vi "Segment_b.vi"(11 "Input in Binary":bool[](array[boolean])) -> (3 "Segment b":bool)   [LabVIEW 2024]
panel:
  out "D":bool
  out "C":bool
  out "B":bool
  out "A":bool
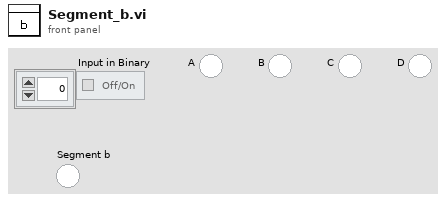
[diagram p1: front panel]
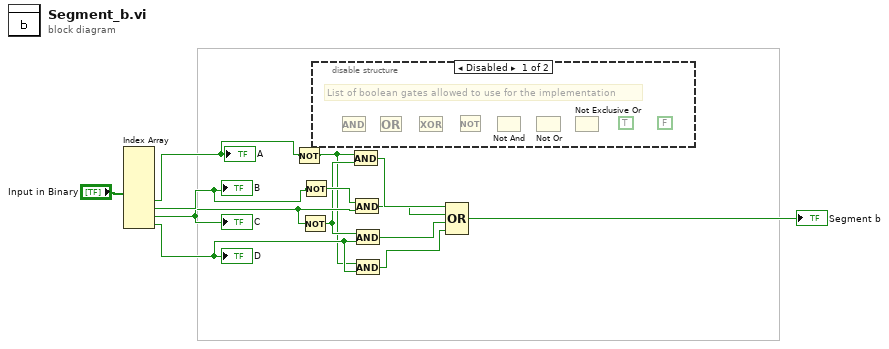
[diagram p0: block diagram]
diagram:
  n1 = Index Array(array="Input in Binary") -> (element #5=w9:bool, element #6=w12:bool, element #7=w10:bool, element #8=w7:bool)  [unwired: 8 in, 4 out]
  "A" <- w9
  "B" <- w12
  "C" <- w10
  "D" <- w7
  n2 = Not(x=w9) -> (.not. x?=w6:bool)
  n3 = Not(x=w10) -> (.not. x?=w8:bool)
  n4 = Not(x=w12) -> (.not. x?=w11:bool)
  n5 = disable-structure shown="Disabled" {
    frame Disabled {
      (unwired) FALSE
      (unwired) TRUE
      # "List of boolean gates allowed to use for the implementation"
      n6 = And() -> ()  [unwired: 2 in, 1 out]
      n7 = Or() -> ()  [unwired: 2 in, 1 out]
      n8 = Exclusive Or() -> ()  [unwired: 2 in, 1 out]
      n9 = Not() -> ()  [unwired: 1 in, 1 out]
      n10 = Not And() -> ()  [unwired: 2 in, 1 out]
      n11 = Not Or() -> ()  [unwired: 2 in, 1 out]
      n12 = Not Exclusive Or() -> ()  [unwired: 2 in, 1 out]
    }
    frame Enabled {
    }
  }
  n13 = And(x=w6, y=w8) -> (x .and. y?=w4:bool)
  n14 = And(x=w11, y=w10) -> (x .and. y?=w3:bool)
  n15 = And(x=w8, y=w7) -> (x .and. y?=w2:bool)
  n16 = And(x=w6, y=w7) -> (x .and. y?=w1:bool)
  n17 = Compound Arithmetic op=OR(w4, w3, w2, w1) -> (→"Segment b":bool)
